vi "Read DevID.vi"(8 "error in (no error)":errorcluster, 11 "Generic Init CVT Message in":refnum<class "Generic Init CVT Message.lvclass">) -> (0 "error out":errorcluster, 2 "DevID":string, 3 "Generic Init CVT Message out":refnum<class "Generic Init CVT Message.lvclass">)   [LabVIEW 2014, in "DAQ Device.lvlib" / "Generic Init CVT Message.lvclass"]
uses:
  Generic Init CVT Message.lvclass
  Generic Init CVT Message.lvclass/Generic Init CVT Message.ctl
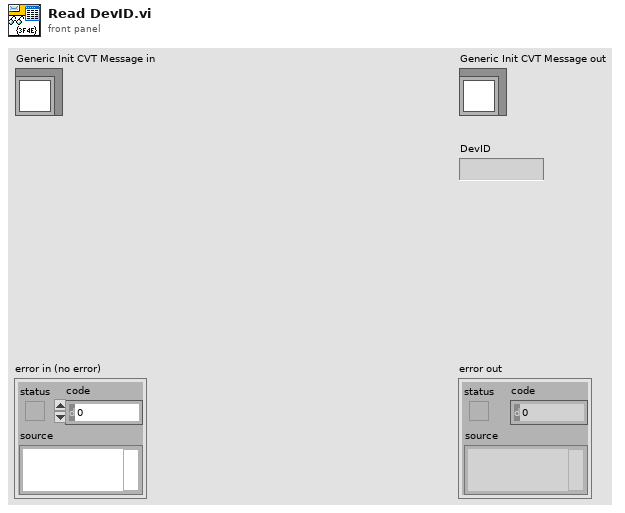
[diagram p1: front panel]
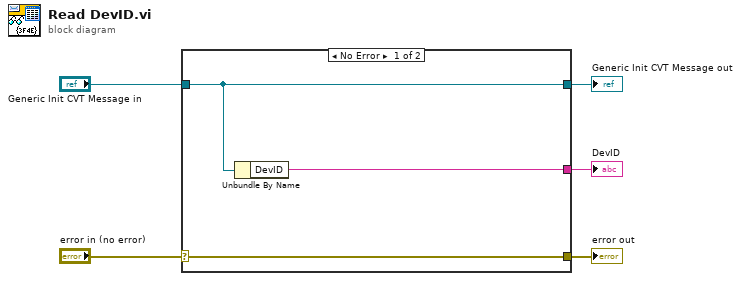
[diagram p0: block diagram]
diagram:
  n1 = case shown="No Error" "error in (no error)" {
    selector: "error in (no error)" -> [w8 w9]
    tunnel: [w8 w9] -> w4
    tunnel: [w7 w10] -> w2
    tunnel: "Generic Init CVT Message in" -> [w7 w10]
    tunnel: [w6 _] -> w1
    frame No Error {
      n2 = Unbundle By Name(w7) -> ("DevID"=w6:string)
    }
    frame Error {
    }
  }
  "error out" <- w4
  "Generic Init CVT Message out" <- w2
  "DevID" <- w1
